vi "生病提醒.vi"(1 "数值":dbl) -> (0 "数值 2":dbl)   [LabVIEW 2018]
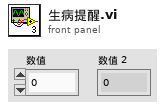
[diagram p1: front panel]
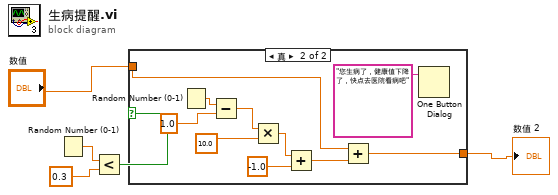
[diagram p0: block diagram]
diagram:
  n1 = Random Number (0-1)() -> (number: 0 to 1=w3:dbl)
  n2 = Less?(x=w3, y=0.3) -> (x < y?=w5:bool)
  n3 = case shown="真" w5 {
    tunnel: [w6 w7] -> w2
    tunnel: "数值" -> [w6 w12]
    frame False {
    }
    frame True {
      n4 = Random Number (0-1)() -> (number: 0 to 1=w15:dbl)
      n5 = Subtract(x=w15, y=1.0) -> (x-y=w14:dbl)
      n6 = Multiply(x=w14, y=10.0) -> (x*y=w10:dbl)
      n7 = Add(x=w10, y=-1.0) -> (x+y=w8:dbl)
      n8 = Add(x=w12, y=w8) -> (x+y=w7:dbl)
      n9 = One Button Dialog(message="您生病了，健康值下降了，快点去医院看病吧" ("姓名输入提示")) -> ()  [unwired: 1 in, 1 out]
    }
  }
  "数值 2" <- w2
